vi "checkFinishPassPlay.vi"(8 "error in (no error)":errorcluster, 10 "Game":refnum<class "Game.lvclass">, 11 "PassPlay in":refnum<class "PassPlay.lvclass">) -> (0 "error out":errorcluster, 2 "Boolean":bool, 3 "PassPlay out":refnum<class "PassPlay.lvclass">)   [LabVIEW 2023, in "PassPlay.lvclass"]
uses:
  PassPlay.lvclass
  Referee_class/command_interpreted.ctl
  Utilities_class/Utilities.lvclass
  Game_class/Game.lvclass
  Events_class/Events.lvclass
  Referee_class/Referee.lvclass
  Enemy_class/Enemy.lvclass
  Ally_class/Ally.lvclass
  Ball_class/Ball.lvclass
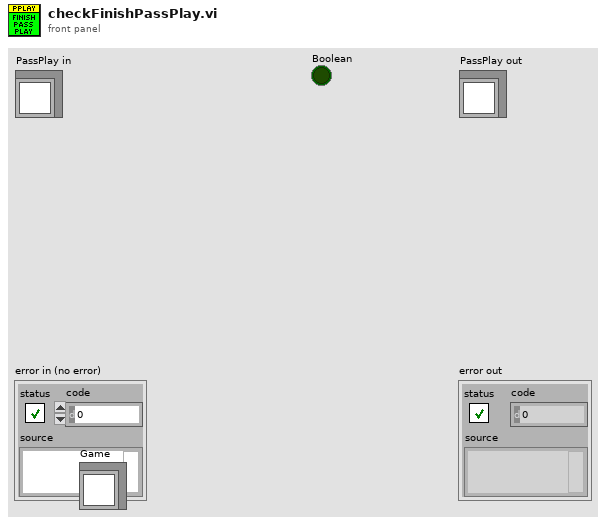
[diagram p1: front panel]
types:
  T1 = typedef "command_interpreted.ctl" = enum16{"Goal Ally", "Goal Enemy", "Ball Placement Enemy", "Ball Placement Ally", "Normal Half Time", "Extra Time  Break", "Extra Half Time", "None", "Post Game", "PKA Normal Start", "Prepare Kickoff Ally", "PKE Normal Start", "Prepare Kickoff Enemy", "Force Start", "Halt", "Timeout", "Prepare Penalty Ally", "Prepare Penalty Enemy", "PPA NormalStart", "PPE Normal Start", "Indirect Free Ally", "Direct Free Enemy", "Direct Free Ally", "Indirect Free Enemy", "Stop"}
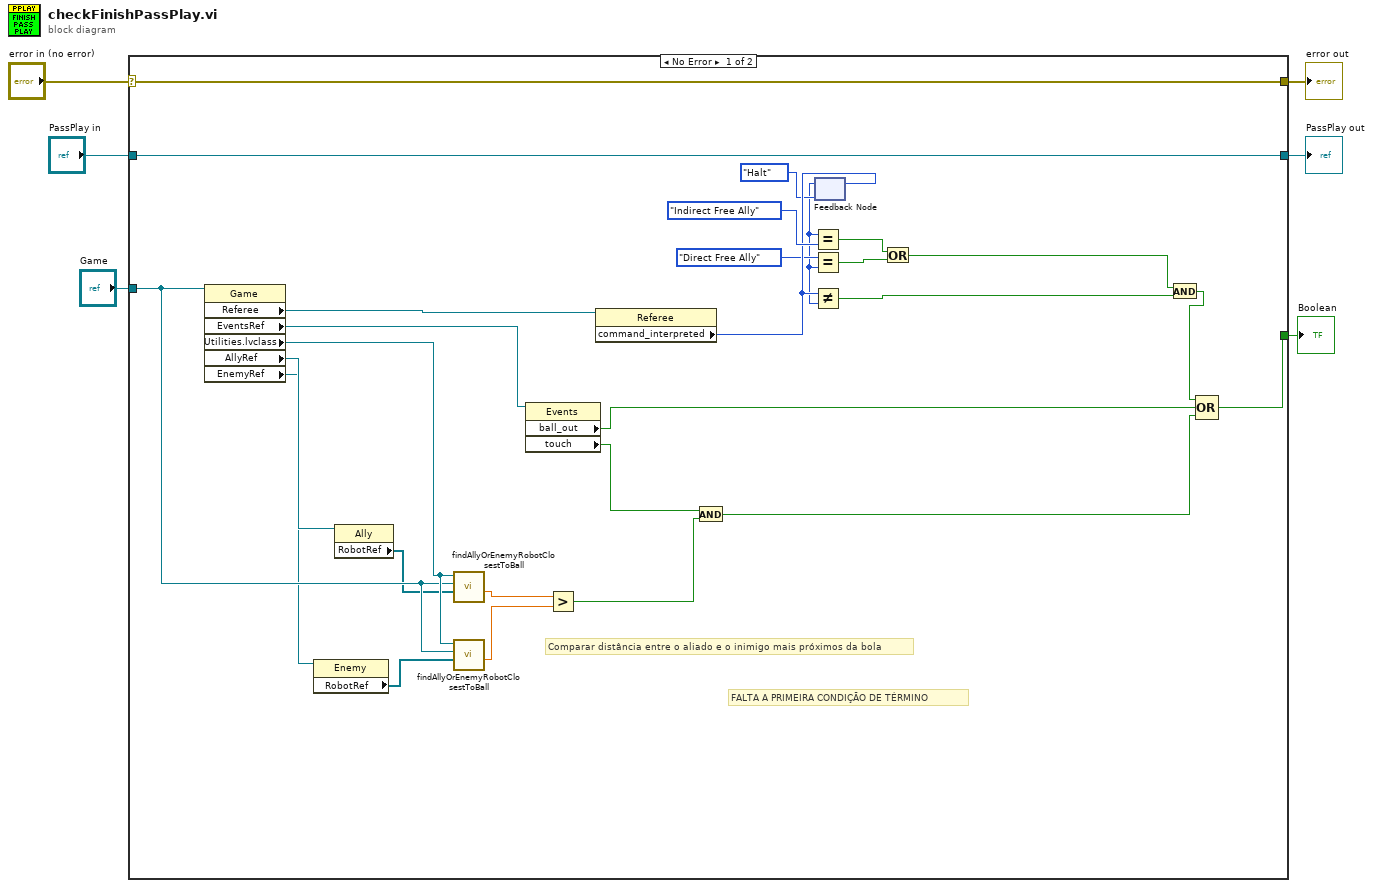
[diagram p0: block diagram]
diagram:
  n1 = case shown="No Error" "error in (no error)" {
    selector: "error in (no error)" -> [w32 w35]
    tunnel: [w32 w35] -> w5
    tunnel: [w33 w34] -> w3
    tunnel: "PassPlay in" -> [w33 w34]
    tunnel: "Game" -> [w16 _]
    tunnel: [w18 _] -> w1
    frame No Error {
      # "Comparar distância entre o aliado e o inimigo mais próximos da bola"
      # "FALTA A PRIMEIRA CONDIÇÃO DE TÉRMINO"
      n2 = property class="Game"(reference=w16) -> ("Referee"=w31:refnum<class "Referee.lvclass">, "EventsRef"=w21:refnum<class "Events.lvclass">, "Utilities.lvclass"=w17:refnum<class "Utilities.lvclass">, "AllyRef"=w15:refnum<class "Ally.lvclass">, "EnemyRef"=w14:refnum<class "Enemy.lvclass">)  [unwired: 1 in, 2 out]
      n3 = property class="Enemy"(reference=w14) -> ("RobotRef"=w12:refnum<class "Robot.lvclass">[])  [unwired: 1 in, 2 out]
      n4 = property class="Ally"(reference=w15) -> ("RobotRef"=w13:refnum<class "Robot.lvclass">[])  [unwired: 1 in, 2 out]
      n5 = call "findAllyOrEnemyRobotClosestToBall.vi"("Ally/Enemy Robots"=w13, "Ball"=w16, "Utilities in"=w17) -> ("Robot distance to ball"=w10:dbl)  [unwired: 5 in, 3 out]
      n6 = call "findAllyOrEnemyRobotClosestToBall.vi"("Ally/Enemy Robots"=w12, "Ball"=w16, "Utilities in"=w17) -> ("Robot distance to ball"=w9:dbl)  [unwired: 5 in, 3 out]
      n7 = property class="Events"(reference=w21) -> ("ball_out"=w19:bool, "touch"=w11:bool)  [unwired: 1 in, 2 out]
      n8 = Greater?(x=w10, y=w9) -> (0:w8:bool)
      n9 = property class="Referee"(reference=w31) -> ("command_interpreted"=w29:T1)  [unwired: 1 in, 2 out]
      n10 = And(x=w11, y=w8) -> (x .and. y?=w7:bool)
      n11 = feedback #1(command_interpreted."Halt" ("command_interpreted")) -> (w25:T1)
      n12 = Equal?(x=w25, y=command_interpreted."Indirect Free Ally" ("command_interpreted")) -> (x = y?=w23:bool)
      n13 = Equal?(x=command_interpreted."Direct Free Ally" ("command_interpreted"), y=w25) -> (x = y?=w24:bool)
      n14 = Not Equal?(x=w29, y=w25) -> (x != y?=w28:bool)
      n15 = feedback-in #1(w29) -> ()
      n16 = Or(x=w23, y=w24) -> (x .or. y?=w22:bool)
      n17 = And(x=w22, y=w28) -> (x .and. y?=w20:bool)
      n18 = Compound Arithmetic op=OR(w20, w19, w7) -> (w18:bool)
    }
    frame Error {
    }
  }
  "error out" <- w5
  "PassPlay out" <- w3
  "Boolean" <- w1
